vi "LogReportError.vi"(8 "error in (no error)":errorcluster) -> (0 "error out":errorcluster)   [LabVIEW 2020]
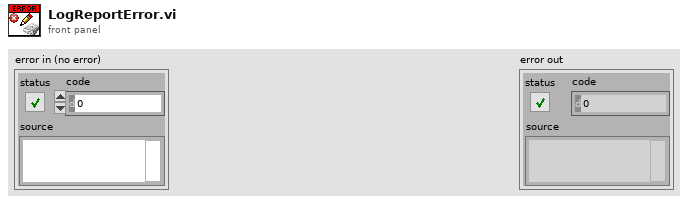
[diagram p1: front panel]
types:
  T1 = enum16{"open", "replace", "create", "open or create", "replace or create", "replace or create with confirmation"}
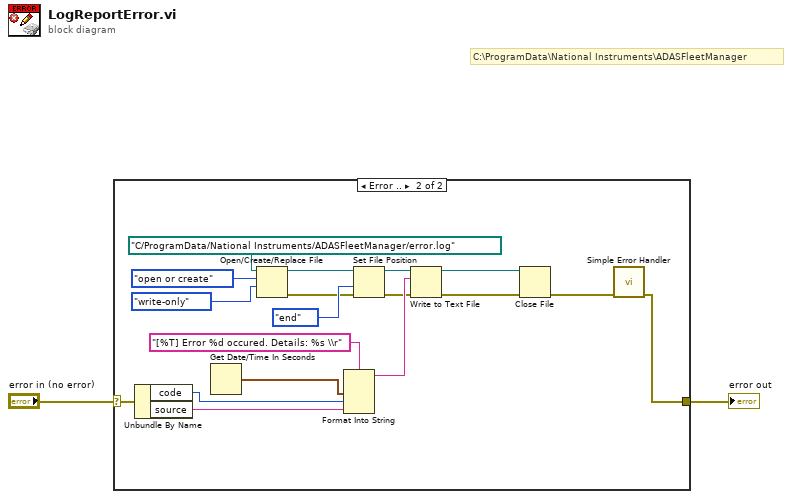
[diagram p0: block diagram]
diagram:
  # "C:\\ProgramData\\National Instruments\\ADASFleetManager"
  n1 = case shown="Error .." "error in (no error)" {
    selector: "error in (no error)" -> [w3 w18]
    tunnel: [w3 w9] -> w1
    frame No Error {
    }
    frame Error {
      n2 = Unbundle By Name(w18) -> ("code"=w16:i32, "source"=w15:string)
      n3 = Get Date/Time In Seconds() -> (seconds since 1Jan1904=w14:timestamp)
      n4 = Open/Create/Replace File(file path (use dialog)=path "C:/ProgramData/National Instruments/ADASFleetManager/error.log", operation (0:open)=T1."open or create", access (0:read/write)=enum16{"read/write", "read-only", "write-only"}."write-only") -> (refnum out=w5:refnum<file>, error out=w7:errorcluster)  [unwired: 3 in, 1 out]
      n5 = Format Into String(format string="[%T] Error %d occured. Details: %s \\r", w14, w16, w15) -> (resulting string=w13:string)  [unwired: 2 in, 1 out]
      n6 = Set File Position(refnum=w5, from (0:start)=enum16{"start", "end", "current"}."end", error in=w7) -> (refnum out=w4:refnum<file>, error out=w6:errorcluster)  [unwired: 1 in]
      n7 = Write to Text File(file (use dialog)=w4, text=w13, error in=w6) -> (refnum out=w11:refnum<file>, error out=w12:errorcluster)  [unwired: 1 in, 1 out]
      n8 = Close File(refnum=w11, error in=w12) -> (error out=w10:errorcluster)  [unwired: 1 out]
      n9 = call <vilib>:"Simple Error Handler.vi"("error in (no error)"=w10) -> ("error out"=w9:errorcluster)  [unwired: 4 in, 4 out]
    }
  }
  "error out" <- w1
